vi "set_input_configuration.vi"(8 "error in (no error)":errorcluster, 9 "Thermocouple type":T2="1", 10 "Sensor type":T1="0", 11 "connection ID":refnum<k5>) -> (0 "error out":errorcluster, 3 "connection ID out":refnum<k5>)   [LabVIEW 2018]
uses:
  typedefs/thermocouple_types.ctl
  typedefs/sensor_types.ctl
panel:
  out "bytes written":i32
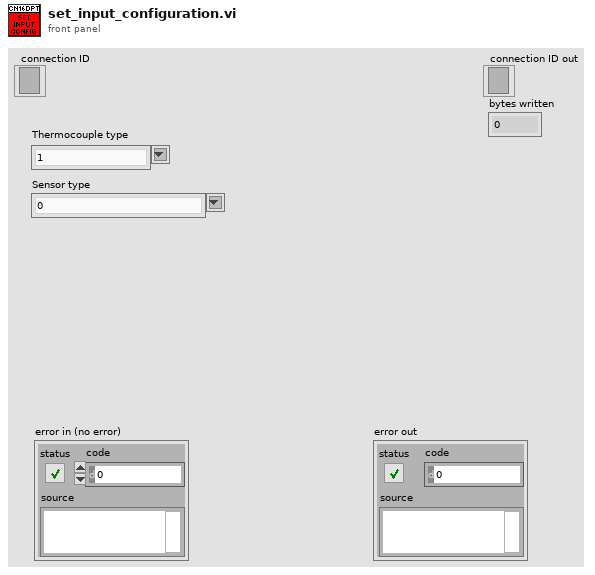
[diagram p1: front panel]
types:
  T1 = typedef "sensor_types.ctl" = string
  T2 = typedef "thermocouple_types.ctl" = string
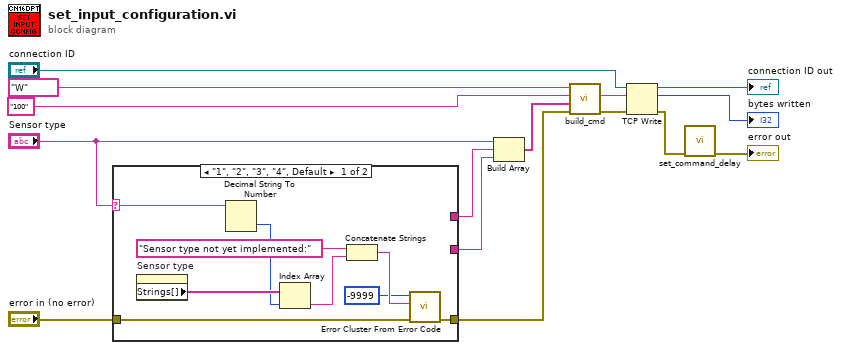
[diagram p0: block diagram]
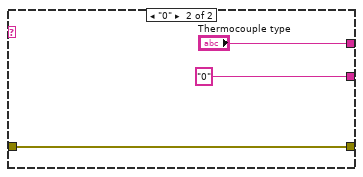
[diagram p2: hidden frame]
diagram:
  n1 = case shown="\"1\", \"2\", \"3\", \"4\", Default" "Sensor type" {
    selector: "Sensor type" -> [w18 _]
    tunnel: [_ "Thermocouple type"] -> w5
    tunnel: [_ "0" ("element")] -> w4
    tunnel: "error in (no error)" -> [w24 w25]
    tunnel: [w23 w25] -> w1
    frame "1", "2", "3", "4", Default {
      n2 = property on="Sensor type" class="CmbBox (strict)"() -> ("Strings[]"=w19:string[])  [unwired: 2 in, 2 out]
      n3 = Decimal String To Number(string=w18) -> (number=w17:i32)  [unwired: 2 in, 1 out]
      n4 = Index Array(array=w19, index=w17) -> (element=w16:string)
      n5 = Concatenate Strings("Sensor type not yet implemented:", w16) -> (w21:string)
      n6 = call <vilib>:"Error Cluster From Error Code.vi"("error in (no error)"=w24, "error message (\"\")"=w21, "error code (0)"=-9999) -> ("error out"=w23:errorcluster)  [unwired: 6 in]
    }
    frame "0" {
    }
  }
  n7 = Build Array("Sensor type", w5, w4) -> (w15:T2[])
  n8 = call "build_cmd.vi"("error in (no error)"=w1, "Parameter list"=w15, "Command ID"="100", "Command class"="W") -> ("error out"=w12:errorcluster, "Command"=w11:string)  [unwired: 6 in]
  n9 = TCP Write(connection ID="connection ID", data in=w11, error in (no error)=w12) -> (connection ID out=→"connection ID out":refnum<k5>, bytes written=→"bytes written":i32, error out=w7:errorcluster)  [unwired: 1 in]
  n10 = call "set_command_delay.vi"("error in (no error)"=w7) -> ("error out"=→"error out":errorcluster)  [unwired: 10 in]
